vi "Log.RetrievePaths.vi"(8 "error in (no error)":errorcluster, 11 "VeriStand Version (2013 SP1)":string) -> (0 "error out":errorcluster, 3 "TestStand Install Directory":string)   [LabVIEW 2014]
uses:
  <vilib>/Utility/sysdir.llb/System Directory Type.ctl
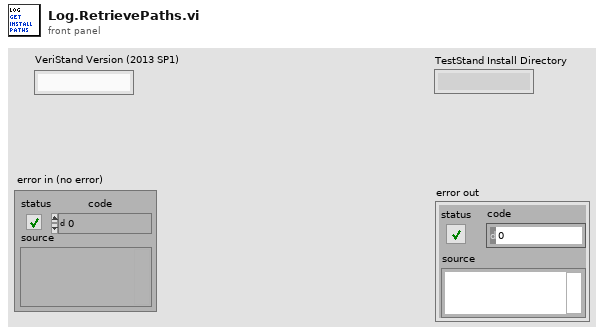
[diagram p1: front panel]
types:
  T1 = enum16{"open", "replace", "create", "open or create", "replace or create", "replace or create with confirmation"}
  T2 = typedef "System Directory Type.ctl" = i32
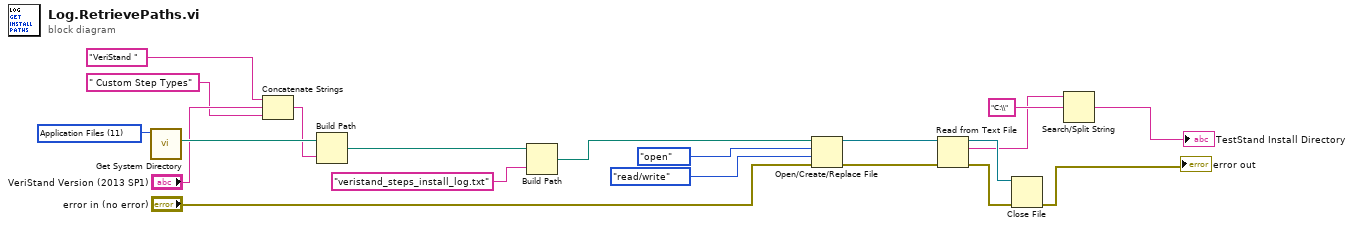
[diagram p0: block diagram]
diagram:
  w20 = T2 11 items=["User Home"=0, "User Desktop"=1, "User Documents"=2, "User Application Data"=3, "User Preferences"=4, "User Temporary"=5, "Public Documents"=6, "Public Application Data"=7, "Public Preferences"=8, "Public Cache"=13, "System Core Libraries"=9, "System Installed Libraries"=10, "Application Files"=11, "Boot Volume Root"=12] ("system directory type")
  n1 = call <vilib>:"Get System Directory.vi"("system directory type"=w20) -> ("system directory"=w19:path)  [unwired: 10 in]
  n2 = Concatenate Strings("VeriStand ", "VeriStand Version (2013 SP1)", " Custom Step Types") -> (w17:string)
  n3 = Build Path(base path=w19, name or relative path=w17) -> (appended path=w9:path)
  n4 = Build Path(base path=w9, name or relative path="veristand_steps_install_log.txt") -> (appended path=w7:path)
  n5 = Open/Create/Replace File(file path (use dialog)=w7, error in="error in (no error)", operation (0:open)=T1."open", access (0:read/write)=enum16{"read/write", "read-only", "write-only"}."read/write") -> (refnum out=w14:refnum<file>, error out=w13:errorcluster)  [unwired: 2 in, 1 out]
  n6 = Read from Text File(file (use dialog)=w14, error in=w13) -> (refnum out=w11:refnum<file>, text=w4:string, error out=w12:errorcluster)  [unwired: 2 in, 1 out]
  n7 = Close File(refnum=w11, error in=w12) -> (error out=→"error out":errorcluster)  [unwired: 1 out]
  n8 = Search/Split String(string=w4, search string/char (-)="C:\\" ("name or relative path")) -> (match + rest of string=→"TestStand Install Directory":string)  [unwired: 1 in, 2 out]
